vi "BSL Flash.vi"(8 "error in":errorcluster, 11 "Notifier in":refnum<notifier>) -> (0 "error out":errorcluster, 3 "Notifier out":refnum<notifier>)   [LabVIEW 2017]
uses:
  controls/FGV DO.ctl
  GV/Towerlight GV.vi
panel:
  out "error out 2":errorcluster
  out "path":path
  # "C:\\DATA\\PROJECTS\\1929 - AAP WR PY1B\\Software\\Software 2020.07.31 1726\\PY1B EOL Integration (2017 32-Bit)\\User Application"
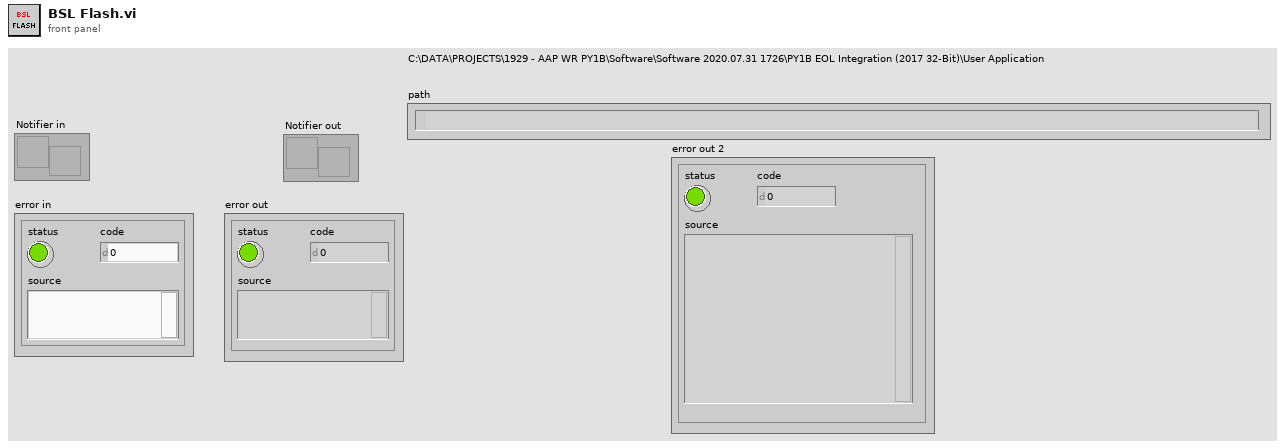
[diagram p1: front panel]
types:
  T1 = typedef "FGV DO.ctl" = enum16{"Initialize", "Start Task", "Clamping", "Load CYL", "Contactors", "Loadcell CYL", "BSL", "Read DO", "Clear Tasks", "Clear Task"}
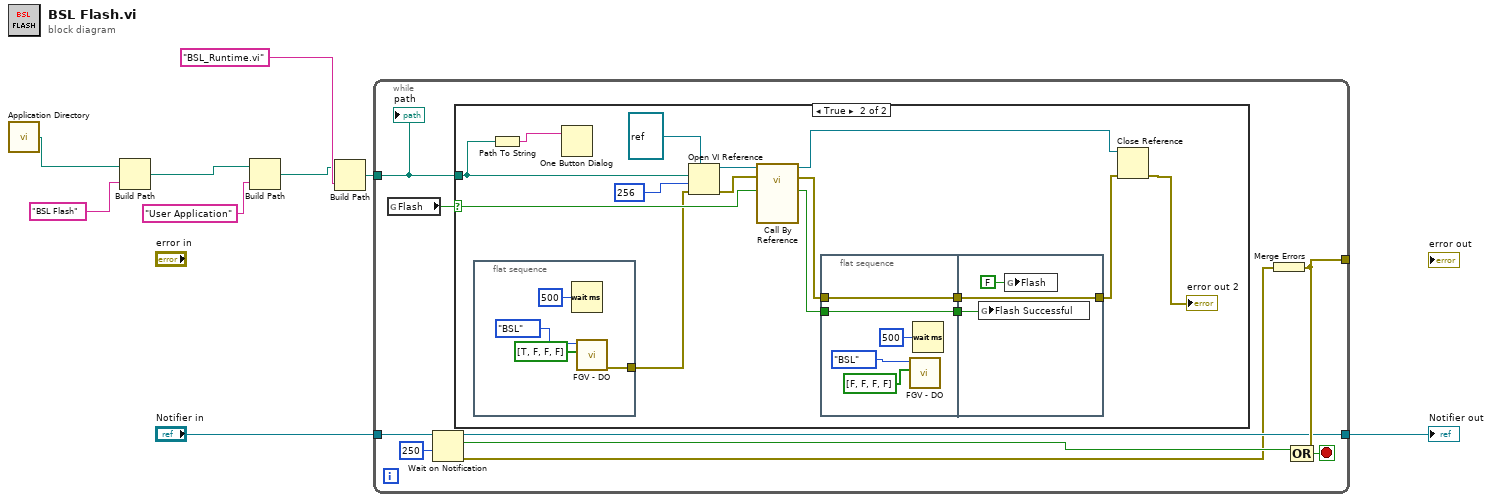
[diagram p0: block diagram]
diagram:
  n1 = call <vilib>:"Application Directory.vi"() -> ("Application Directory"=w4:path)
  n2 = Build Path(base path=w4, name or relative path="BSL Flash") -> (appended path=w3:path)
  n3 = Build Path(base path=w3, name or relative path="User Application") -> (appended path=w2:path)
  n4 = Build Path(base path=w2, name or relative path="BSL_Runtime.vi") -> (appended path=w5:path)
  n5 = while {
    tunnel: [w17] -> _
    tunnel: "Notifier in" -> [w16]
    tunnel: [w13] -> w8
    tunnel: w5 -> [w10]
    stop <- w18 stop-if-true
    n6 = global read "Towerlight GV.vi" "Flash"() -> (w11:bool)
    n7 = Wait on Notification(notifier=w16, timeout in ms (-1)=250) -> (notifier out=w13:refnum<notifier>, notification=w14:bool, error out=w12:errorcluster)  [unwired: 2 in, 1 out]
    n8 = case shown="True" w11 {
      selector: w11 -> [_ w32]
      tunnel: w10 -> [_ w22]
      frame False {
      }
      frame True {
        n9 = flat-sequence {
          tunnel: [w35] -> w25
          frame #0 {
            n10 = Wait (ms)(milliseconds to wait=u32 500) -> ()  [unwired: 1 out]
            n11 = call "FGV - DO.vi"("Digital Outs"=bool[] [TRUE, FALSE, FALSE, FALSE], "State"=FGV_DO."BSL") -> ("error out"=w35:errorcluster)  [unwired: 8 in, 1 out]
          }
        }
        n12 = Path To String(path=w22) -> (string=w21:string)
        n13 = One Button Dialog(message=w21) -> ()  [unwired: 1 in, 1 out]
        n14 = Open VI Reference(type specifier VI Refnum (for type only)=refnum<vi> refnum, vi path=w22, options=256, error in (no error)=w25) -> (vi reference=w33:refnum<vi>, error out=w29:errorcluster)  [unwired: 2 in]
        n15 = call-by-ref "?"(reference=w33, error in=w29, "Auto-Execution Control"=w32) -> (reference out=w27:refnum<vi>, error out=w31:errorcluster, "Auto execution status"=w30:bool)  [unwired: 10 in]
        n16 = flat-sequence {
          tunnel: w30 -> [w41]
          tunnel: w31 -> [w42]
          tunnel: [w42] -> w24
          tunnel: [w41] -> w23
          tunnel: [w43] -> w26
          tunnel: w24 -> [w43]
          tunnel: w23 -> [w44]
          frame #0 {
            n17 = call "FGV - DO.vi"("Digital Outs"=bool[] [FALSE, FALSE, FALSE, FALSE], "State"=FGV_DO."BSL") -> ()  [unwired: 8 in, 2 out]
            n18 = Wait (ms)(milliseconds to wait=u32 500) -> ()  [unwired: 1 out]
          }
          frame #1 {
            n19 = global write "Towerlight GV.vi" "Flash Successful"(w44) -> ()
            n20 = global write "Towerlight GV.vi" "Flash"(FALSE ("Flash")) -> ()
          }
        }
        n21 = Close Reference(reference=w27, error in (no error)=w26) -> (error out=→"error out 2":errorcluster)
      }
    }
    n22 = Merge Errors(w12) -> (w17:errorcluster)
    n23 = Compound Arithmetic op=OR(w14, w17) -> (w18:bool)
    "path" <- w10
  }
  "Notifier out" <- w8
